vi "DumbDash Load Values.vi"(7 "Message Box":refnum<vi>, 11 "Controls In":T1[](array[typedef])) -> ()   [LabVIEW 2015]
uses:
  DumbDash Control.ctl
  DumbDash Control Type.ctl
  <vilib>/Utility/sysdir.llb/System Directory Type.ctl
  <vilib>/Utility/config.llb/Read Key (Double).vi
  <vilib>/Utility/config.llb/Read Key (Boolean).vi
  <vilib>/Utility/config.llb/Read Key (String).vi
  <vilib>/Utility/config.llb/NI_LVConfig.lvlib
panel:
  out "file path":path
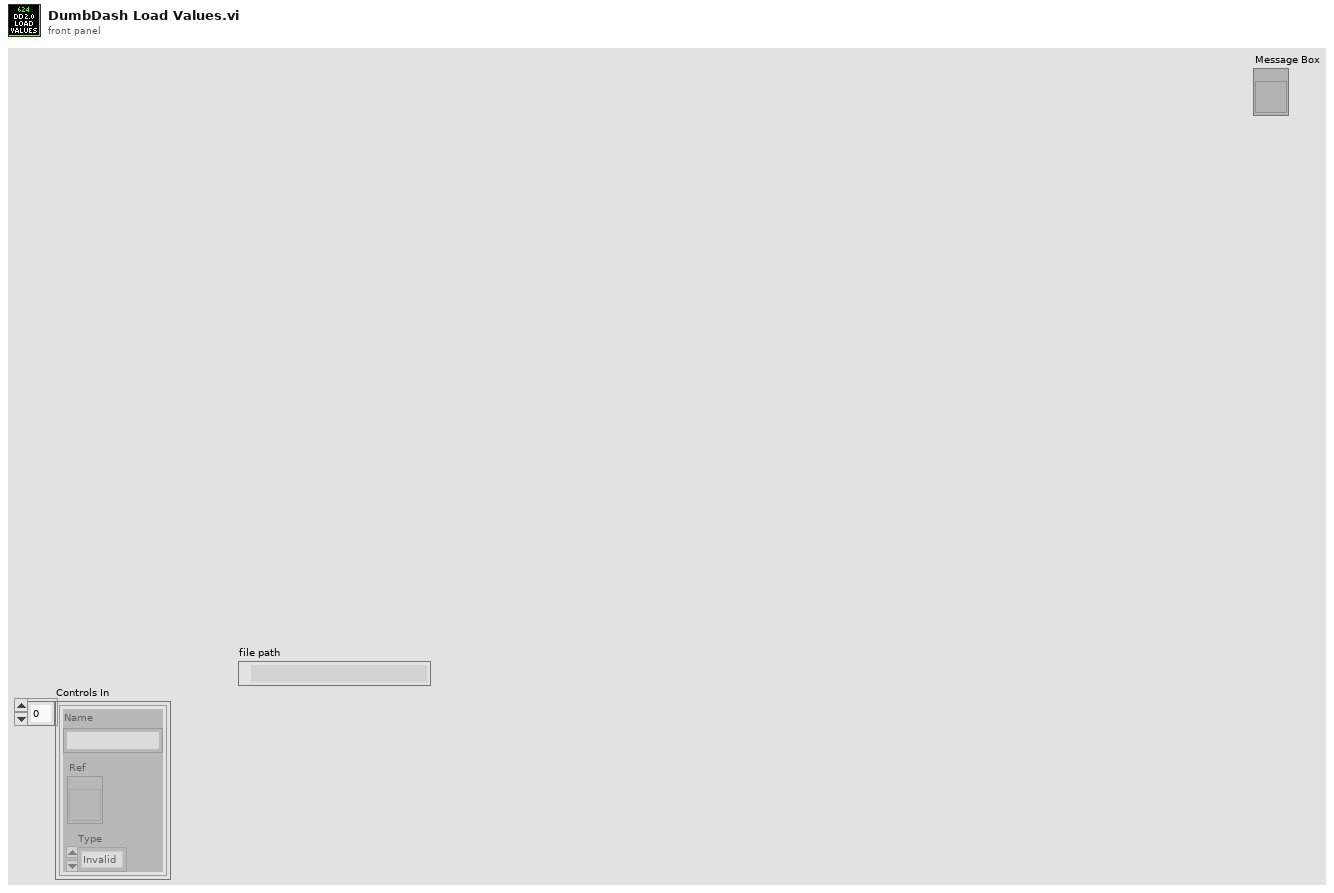
[diagram p1: front panel]
types:
  T1 = typedef "DumbDash Control.ctl" = cluster{"Name":string, "Ref":refnum<vi>, "Type":T2}
  T2 = typedef "DumbDash Control Type.ctl" = enum16{"Invalid", "Number", "Boolean", "String"}
  T3 = typedef "System Directory Type.ctl" = i32
  T4 = typedef "NI_LVConfig.lvlib/Config Data RefNum.ctl" = refnum<k1>
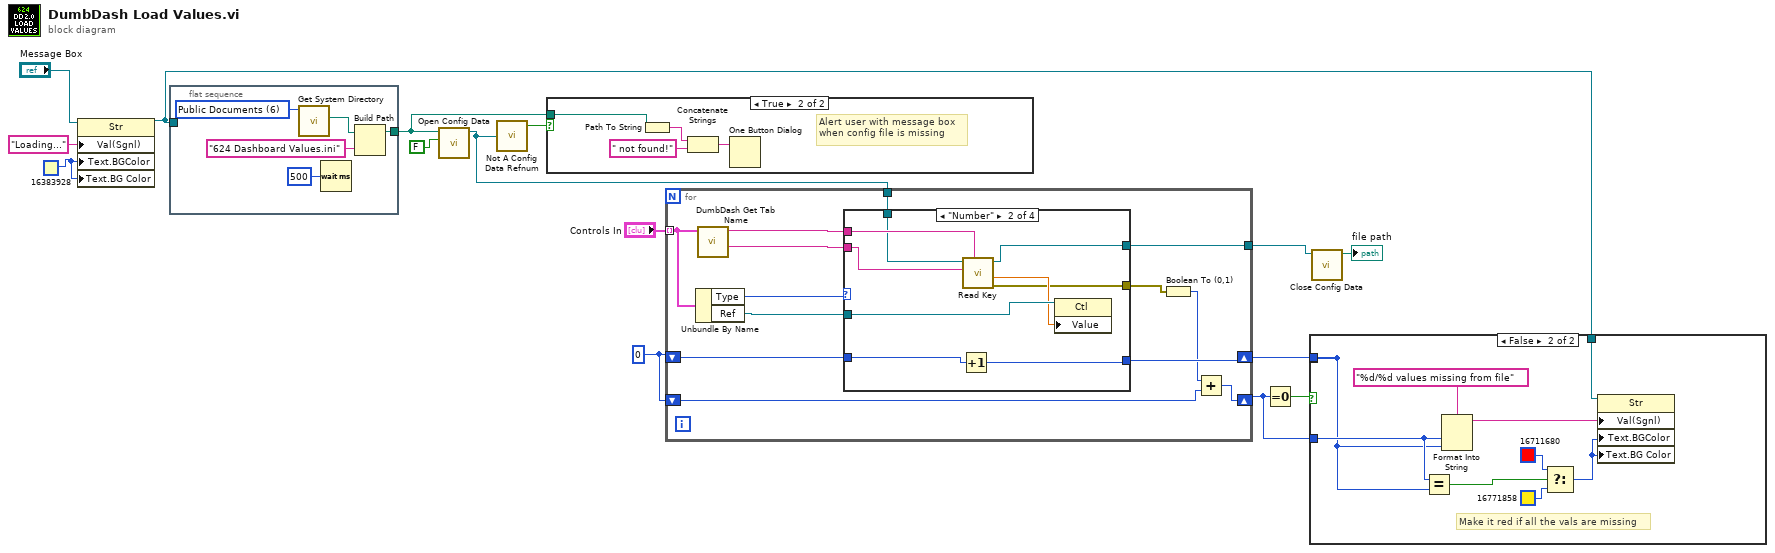
[diagram p0: block diagram]
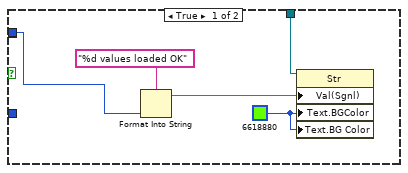
[diagram p3: hidden frame]
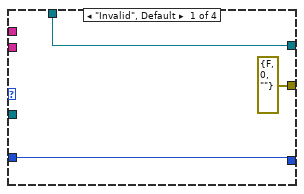
[diagram p4: hidden frame]
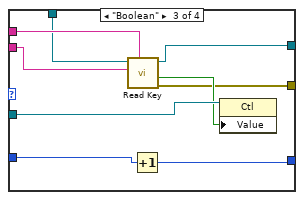
[diagram p5: hidden frame]
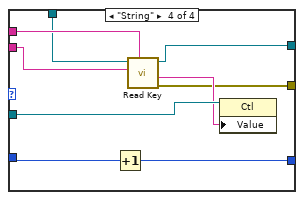
[diagram p6: hidden frame]
diagram:
  w8 = 0
  w9 = u32 16383928
  n1 = property class="Str"(reference="Message Box", "Val(Sgnl)"="Loading..." ("Text.Text"), "Text.BGColor"=w9, "Text.BG Color"=w9) -> (reference out=w4:refnum<vi>)  [unwired: 1 in, 1 out]
  n2 = flat-sequence {
    tunnel: [w17] -> w1
    tunnel: w4 -> [_]
    frame #0 {
      w20 = T3 6 items=["User Home"=0, "User Desktop"=1, "User Documents"=2, "User Application Data"=3, "User Preferences"=4, "User Temporary"=5, "Public Documents"=6, "Public Application Data"=7, "Public Preferences"=8, "Public Cache"=13, "System Core Libraries"=9, "System Installed Libraries"=10, "Application Files"=11, "Boot Volume Root"=12] ("system directory type")
      n3 = call <vilib>:"Get System Directory.vi"("system directory type"=w20) -> ("system directory"=w19:path)  [unwired: 10 in]
      n4 = Wait (ms)(milliseconds to wait=u32 500) -> ()  [unwired: 1 out]
      n5 = Build Path(base path=w19, name or relative path="624 Dashboard Values.ini") -> (appended path=w17:path)
    }
  }
  n6 = call <vilib>:"Open Config Data.vi"("create file if necessary (T)"=FALSE, "configuration file path"=w1) -> ("refnum"=w3:T4)  [unwired: 7 in, 2 out]
  n7 = call <vilib>:"Not A Config Data Refnum.vi"("refnum"=w3) -> ("not a config data refnum"=w2:bool)
  n8 = case shown="True" w2 {
    tunnel: w1 -> [_ w21]
    frame False {
    }
    frame True {
      # "Alert user with message box\nwhen config file is missing"
      n9 = Path To String(path=w21) -> (string=w24:string)
      n10 = Concatenate Strings(w24, " not found!" ("string")) -> (w22:string)
      n11 = One Button Dialog(message=w22) -> ()  [unwired: 1 in, 1 out]
    }
  }
  n12 = for {
    tunnel: "Controls In" -> [w33] mode=indexing
    tunnel: w3 -> [w36]
    tunnel: [w32] -> w14
    shift-right: [w29] -> w6
    shift-left: w8 -> [w30]
    shift-right: [w25] -> w5
    shift-left: w8 -> [w26]
    n13 = Unbundle By Name(w33) -> ("Type"=w34:T2, "Ref"=w31:refnum<vi>)
    n14 = call "DumbDash Get Tab Name.vi"("Cluster"=w33) -> ("Rest of Name"=w35:string, "Tab Name"=w37:string)  [unwired: 9 in]
    n15 = case shown="\"Number\"" w34 {
      tunnel: w37 -> [_ w49 w58 w67]
      tunnel: w36 -> [w40 w48 w57 w66]
      tunnel: w35 -> [_ w47 w56 w65]
      tunnel: [w40 w46 w55 w64] -> w32
      tunnel: w31 -> [_ w45 w54 w63]
      tunnel: w30 -> [w39 w43 w52 w61]
      tunnel: [w39 w42 w51 w60] -> w29
      tunnel: [errorcluster {"status"=FALSE, "code"=0, "source"=""} ("error out") w41 w50 w59] -> w28
      frame "Invalid", Default {
      }
      frame "Number" {
        n16 = Increment(x=w43) -> (x+1=w42:i32)
        n17 = call-poly <vilib>:"Read Key.vi"("section"=w49, "key"=w47, "refnum"=w48) -> ("error out"=w41:errorcluster, "value"=w44:dbl, "refnum out"=w46:T4)  [unwired: 5 in, 1 out]
        n18 = property class="Ctl"(reference=w45, "Value"=w44) -> ()  [unwired: 1 in, 2 out]
      }
      frame "Boolean" {
        n19 = call-poly <vilib>:"Read Key.vi"("section"=w58, "key"=w56, "refnum"=w57) -> ("error out"=w50:errorcluster, "value"=w53:bool, "refnum out"=w55:T4)  [unwired: 5 in, 1 out]
        n20 = Increment(x=w52) -> (x+1=w51:i32)
        n21 = property class="Ctl"(reference=w54, "Value"=w53) -> ()  [unwired: 1 in, 2 out]
      }
      frame "String" {
        n22 = Increment(x=w61) -> (x+1=w60:i32)
        n23 = call-poly <vilib>:"Read Key.vi"("section"=w67, "key"=w65, "refnum"=w66) -> ("error out"=w59:errorcluster, "value"=w62:string, "refnum out"=w64:T4)  [unwired: 5 in, 1 out]
        n24 = property class="Ctl"(reference=w63, "Value"=w62) -> ()  [unwired: 1 in, 2 out]
      }
    }
    n25 = Boolean To (0,1)(Boolean=w28) -> (0, 1=w27:i16)
    n26 = Add(x=w27, y=w26) -> (x+y=w25:i32)
  }
  n27 = Equal To 0?(x=w5) -> (x = 0?=w7:bool)
  n28 = case shown="False" w7 {
    tunnel: [w69 w77] -> _
    tunnel: w6 -> [w69 w77]
    tunnel: w5 -> [_ w78]
    tunnel: w4 -> [w68 w79]
    frame True {
      w70 = u32 6618880
      n29 = Format Into String(format string="%d values loaded OK", w69) -> (resulting string=w71:string)  [unwired: 2 in, 1 out]
      n30 = property class="Str"(reference=w68, "Val(Sgnl)"=w71, "Text.BGColor"=w70, "Text.BG Color"=w70) -> ()  [unwired: 1 in, 2 out]
    }
    frame False {
      # "Make it red if all the vals are missing"
      n31 = Equal?(x=w78, y=w77) -> (x = y?=w76:bool)
      n32 = Format Into String(format string="%d/%d values missing from file", w78, w77) -> (resulting string=w80:string)  [unwired: 2 in, 1 out]
      n33 = Select(t=u32 16711680, s=w76, f=u32 16771858) -> (s? t:f=w73:u32)
      n34 = property class="Str"(reference=w79, "Val(Sgnl)"=w80, "Text.BGColor"=w73, "Text.BG Color"=w73) -> ()  [unwired: 1 in, 2 out]
    }
  }
  n35 = call <vilib>:"Close Config Data.vi"("refnum"=w14) -> ("file path"=→"file path":path)  [unwired: 9 in, 1 out]
